vi "Open_LoopTesting_VI.vi"() -> ()   [LabVIEW 2022 SP3]
uses:
  <vilib>/DAQmx/read.llb/DAQmx Read (Analog 1D Wfm NChan NSamp).vi
  <vilib>/Analysis/baseanly.llb/Mean (DBL).vi
  STOP_GLOBAL.vi
  <vilib>/DAQmx/configure/timing.llb/DAQmx Timing (Sample Clock).vi
  <vilib>/DAQmx/miscellaneous.llb/DAQmx Fill In Error Info.vi
  <resource>/objmgr/daqmx.rc
  <vilib>/Analysis/NI_AALBase.lvlib
panel:
  out "Angle":dbl
  in  "Voltage 2":dbl
  out "Angle Sensor":dbl[](graph)
  out "Voltage Command Output":dbl[](graph)
  out "VoltageSent":dbl
  out "Ball Valve Angle Command":dynamicdata(graph)
  in  "Ignition":bool
  out "Chamber Pressure LocalVar":dynamicdata(graph)
  out "Process Variable vs Setpoint":dynamicdata(graph)
  out "Servo/Step Voltage":dbl[](array[numeric])
  in  "SP":dbl
  out "MV":dbl(slide)=30.8641975308642 scale=0.0..5.067 scale format="%.1f"
  in  "Stop All":bool
  out "D.C. Delay":dbl
  out "AI7":dynamicdata(graph)
  out "Time":dbl
  out "Inlet Thermocouple":cluster{dbl[], dbl[]}(graph)
  out "Inlet Thermocouple":dynamicdata(graph)
  out "Flow Meter Thermocouple":dynamicdata(graph)
  out "Flow Meter Thermocouple":cluster{dbl[], dbl[]}(graph)
  out "Supply P. Thermocouple":cluster{dbl[], dbl[]}(graph)
  out "Supply P. Thermocouple":dynamicdata(graph)
  out "Thrust 3":cluster{dbl[], dbl[]}(graph)
  out "Thrust 2":cluster{dbl[], dbl[]}(graph)
  out "Rocket Thrust":cluster{dbl[], dbl[]}(graph)
  out "LC2":dynamicdata(graph)
  out "Rocket Thrust LC1":dynamicdata(graph)
  out "LC3":dynamicdata(graph)
  out "Waiting \nfor Start":bool=TRUE
  in  "Start VI":bool
  out "SampClk.Rate":dbl
  in  "Sample Number":i32=100
  in  "Channel Control":bool[](array[boolean])
  in  "Rate":dbl=1000.0 format="%0.2f"
  out "AI7":cluster{dbl[], dbl[]}(graph)
  out "Vol Flow L/min":dynamicdata(graph)
  out "Chamber Pressure and Degrees":cluster{dbl[], dbl[]}[](graph)
  in  "Filename":path=path "C:/1. Rocket Research Project/CollectedData/Plots/TestingData.lvm"
  in  "Collect?":bool=TRUE caption="Enable"
  out "Vol Flow":cluster{dbl[], dbl[]}(graph)
  out "Chamber Pressure":cluster{dbl[], dbl[]}(graph)
  out "Inlet Pressure":cluster{dbl[], dbl[]}(graph)
  out "Flow Meter Pressure":cluster{dbl[], dbl[]}(graph)
  out "Supply Pressure":cluster{dbl[], dbl[]}(graph)
  out "Supply Pressure":dynamicdata(graph)
  out "Inlet Pressure":dynamicdata(graph)
  out "Line Pressure":dynamicdata(graph)
  out "Chamber Pressure PSI":dynamicdata(graph)
  out "Output Clock Rate":dbl
  out "For loop iterations":i32
  out "error out":errorcluster
  out "Iterations":i32
  out "Angle Sensor":dynamicdata(graph)
  out "P.T. 5":dynamicdata(graph)
  # "Temperature Channels"
  # "Thrust Channels"
  # "DAQ Configuration"
  # "AI 0 - Supply Pressure"
  # "AI 1 - Flow Meter Pressure"
  # "AI 2 - Inlet Pressure"
  # "AI 3 - Chamber Pressure"
  # "AI 4 - Differential Pressure"
  # "AI 5 - Volumetric Flow"
  # "AI 6 - Angle Sensor"
  # "AI 7"
  # "Load Cell 1 Right"
  # "Load Cell 2 Left"
  # "Thrust Channel 3"
  # "TC1 - Supply P. Thermocouple"
  # "TC2 - Flow Meter Thermocouple"
  # "TC3 - Inlet Thermocouple"
  # "Pressure Channels"
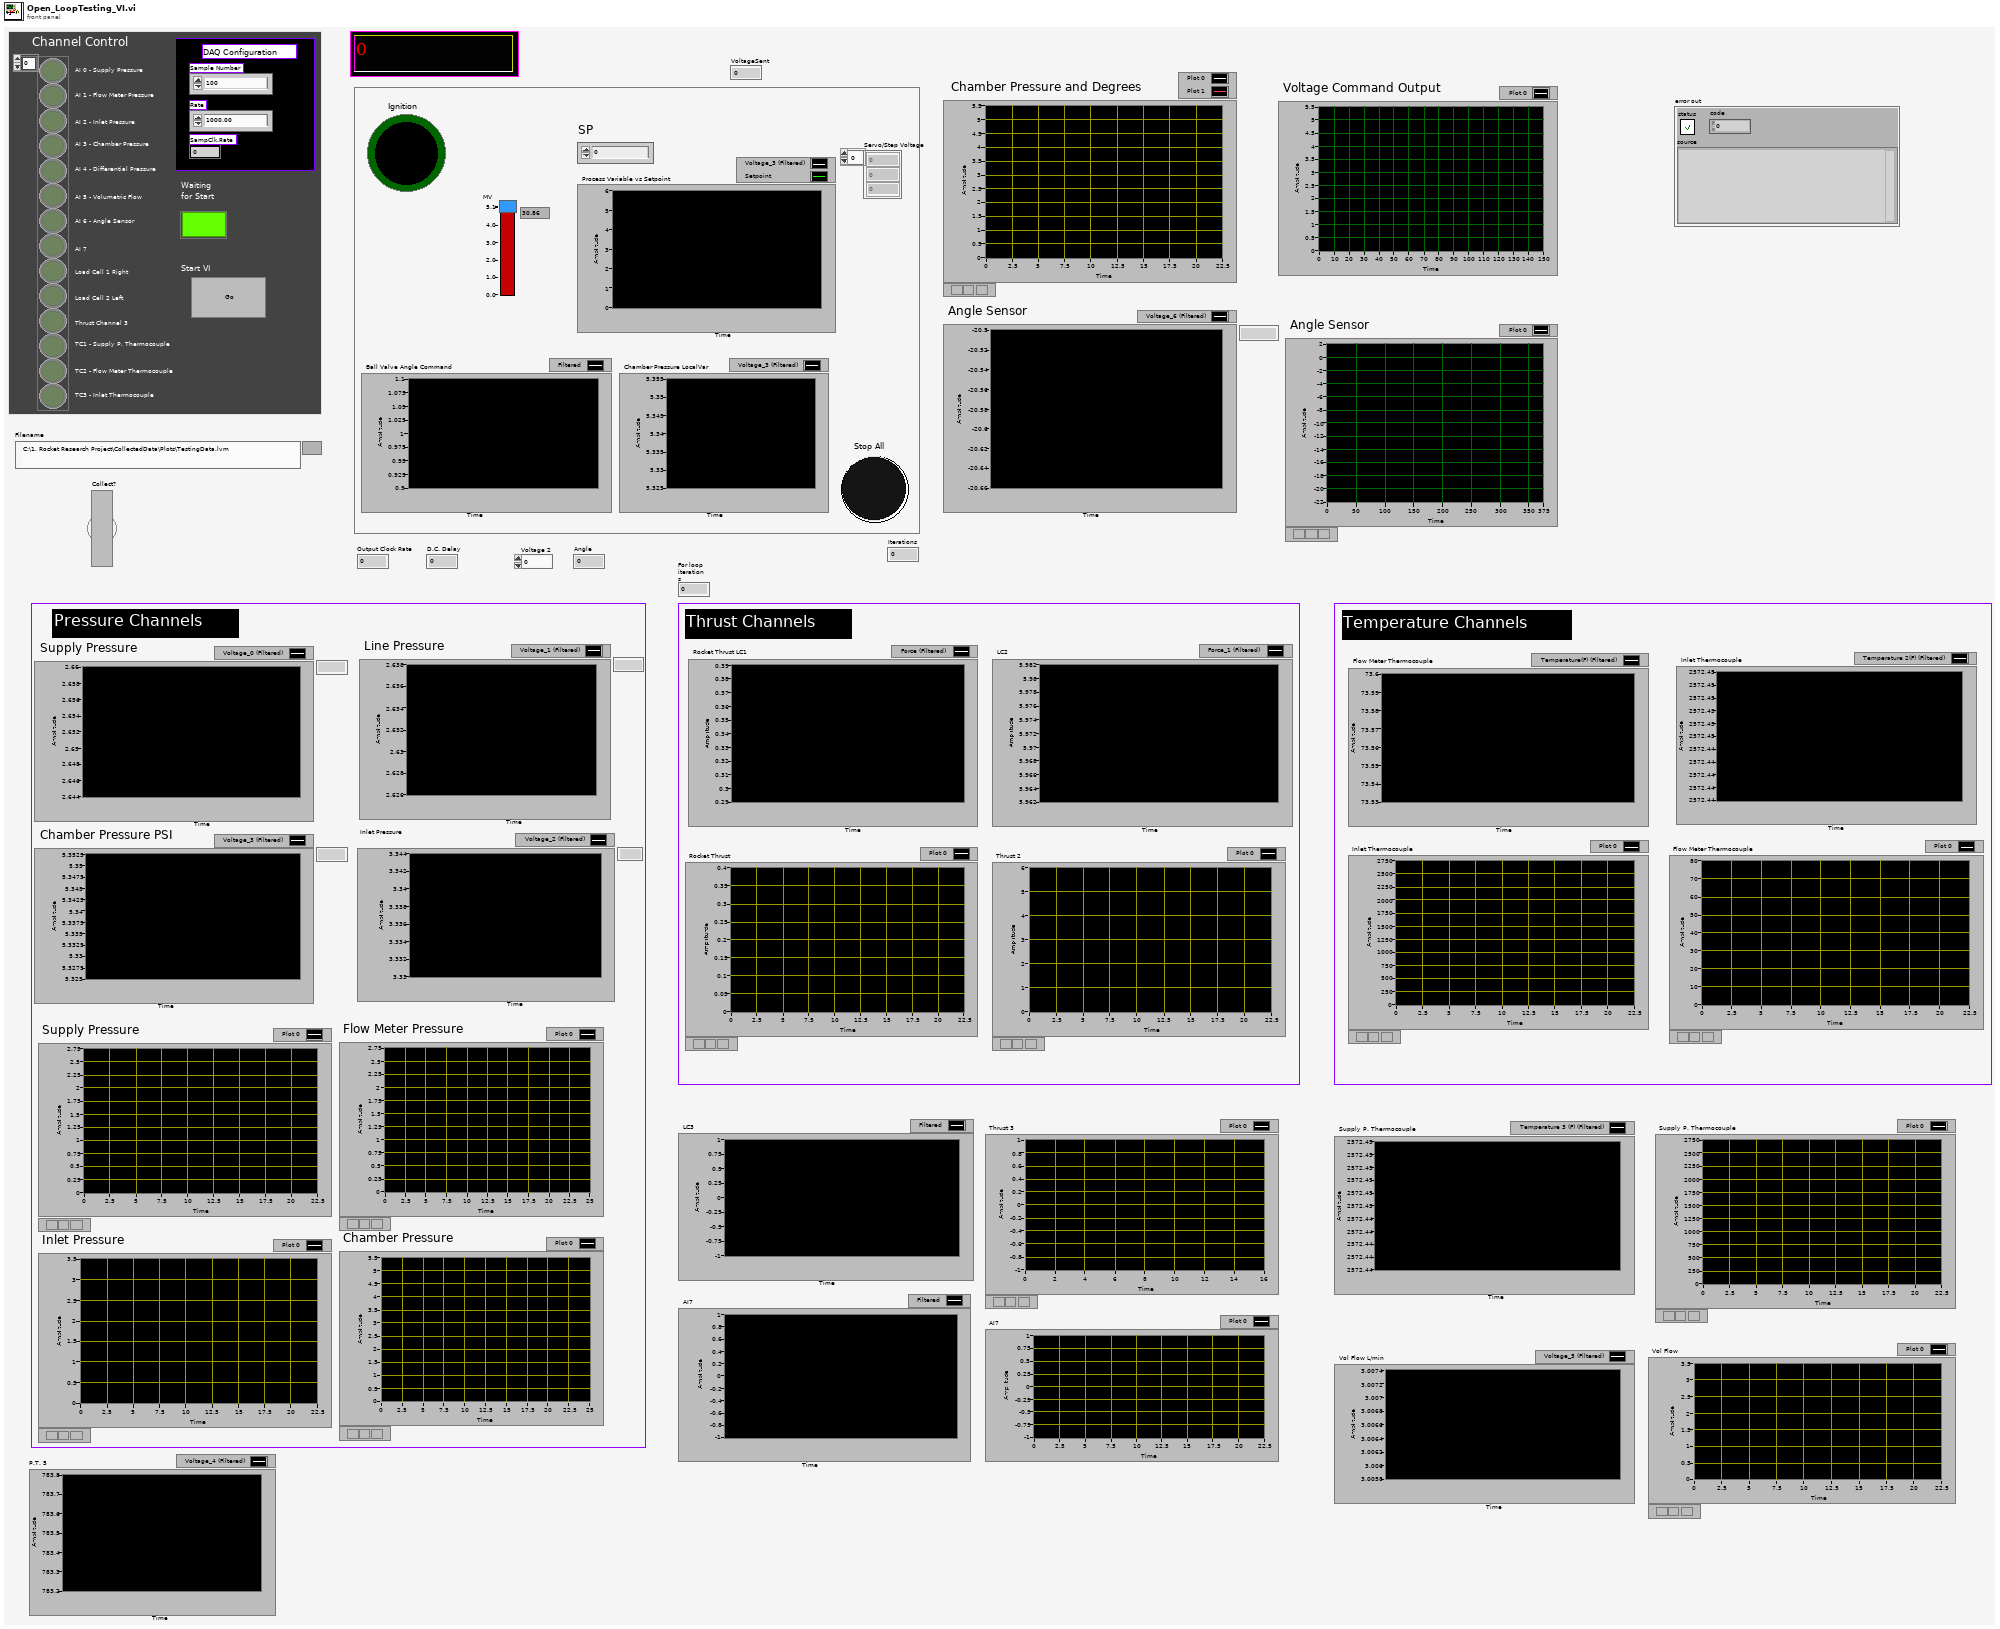
[diagram p1: front panel]
types:
  T1 = cluster{"PID gains":cluster{"Kc":dbl, "Ti":dbl, "Td":dbl}, "max value":dbl}[]
  T2 = cluster{"Modulus":dbl, "Number of\nComplete Cycles":dbl}
  T3 = cluster{"Dynamic Data":dynamicdata, "Dynamic Data":dynamicdata, "Dynamic Data":dynamicdata, "Dynamic Data":dynamicdata, "Dynamic Data":dynamicdata, "Dynamic Data":dynamicdata, "Dynamic Data":dynamicdata, "Dynamic Data":dynamicdata, "Dynamic Data":dynamicdata, "Dynamic Data":dynamicdata, "Dynamic Data":dynamicdata, "Dynamic Data":dynamicdata, "Dynamic Data":dynamicdata, "Dynamic Data":dynamicdata}
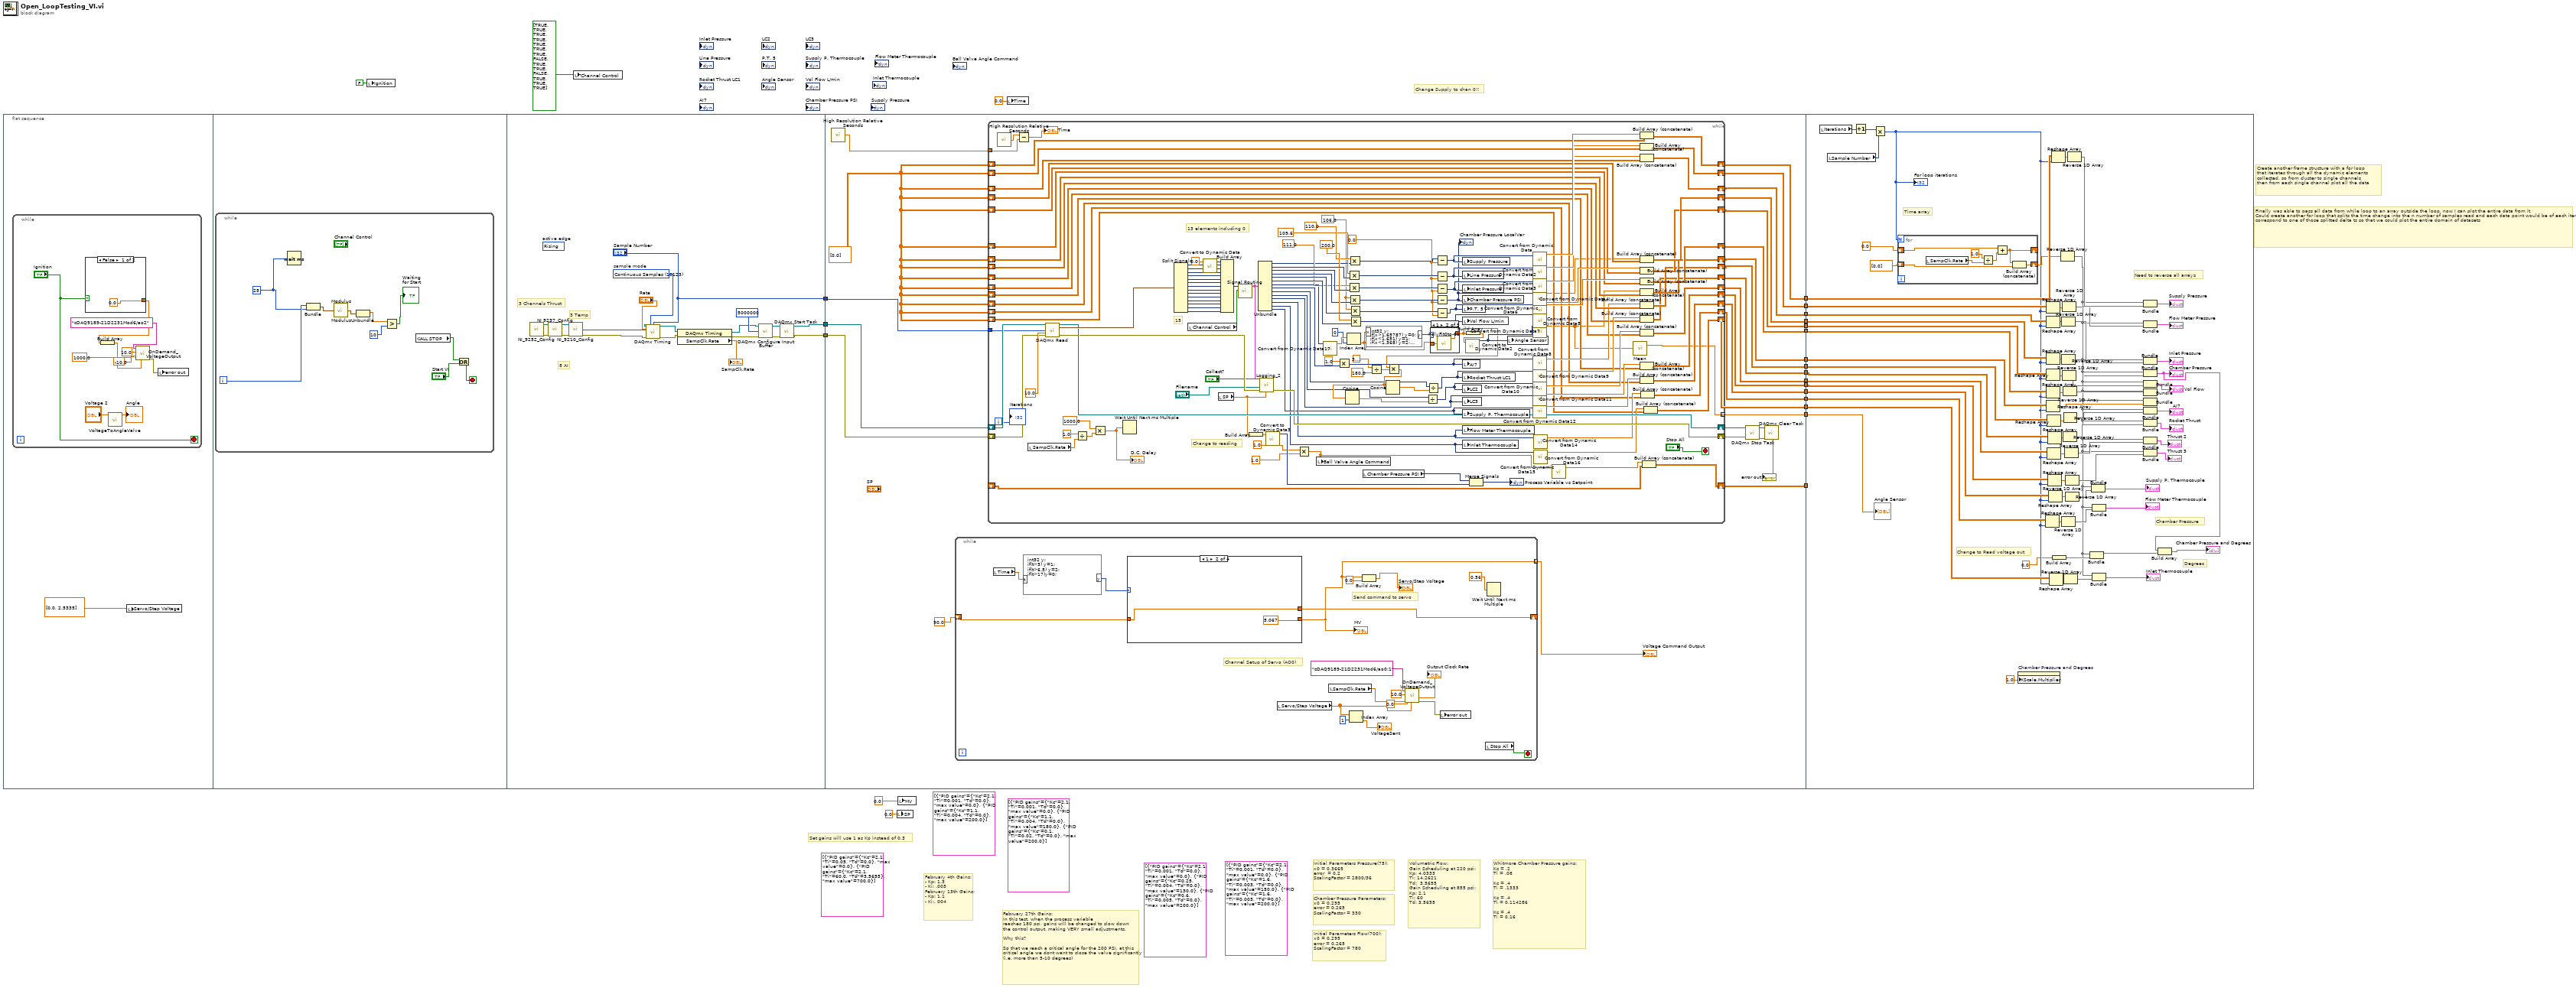
[diagram p0: block diagram]
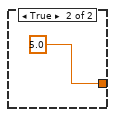
[diagram p2: hidden frame]
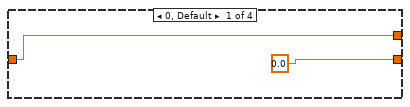
[diagram p3: hidden frame]
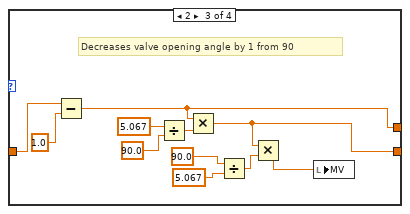
[diagram p4: hidden frame]
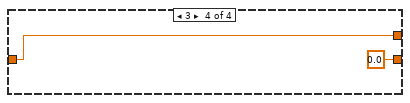
[diagram p5: hidden frame]
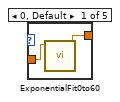
[diagram p6: hidden frame]
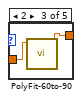
[diagram p7: hidden frame]
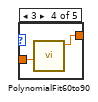
[diagram p8: hidden frame]
diagram:
  (unwired) T1 [{"PID gains"={"Kc"=2.1, "Ti"=0.001, "Td"=0.0}, "max value"=0.0}, {"PID gains"={"Kc"=1.1, "Ti"=0.004, "Td"=0.0}, "max value"=180.0}, {"PID gains"={"Kc"=0.1, "Ti"=0.02, "Td"=0.0}, "max value"=200.0}]
  (unwired) T1 [{"PID gains"={"Kc"=2.1, "Ti"=0.001, "Td"=0.0}, "max value"=0.0}, {"PID gains"={"Kc"=1.6, "Ti"=0.003, "Td"=0.0}, "max value"=150.0}, {"PID gains"={"Kc"=1.6, "Ti"=0.003, "Td"=0.0}, "max value"=200.0}]
  (unwired) T1 [{"PID gains"={"Kc"=2.1, "Ti"=0.001, "Td"=0.0}, "max value"=0.0}, {"PID gains"={"Kc"=0.25, "Ti"=0.004, "Td"=0.0}, "max value"=130.0}, {"PID gains"={"Kc"=0.6, "Ti"=0.005, "Td"=0.0}, "max value"=200.0}]
  (unwired) T1 [{"PID gains"={"Kc"=2.1, "Ti"=0.05, "Td"=0.0}, "max value"=0.0}, {"PID gains"={"Kc"=2.1, "Ti"=60.0, "Td"=3.5655}, "max value"=700.0}]
  (unwired) T1 [{"PID gains"={"Kc"=2.1, "Ti"=0.001, "Td"=0.0}, "max value"=0.0}, {"PID gains"={"Kc"=1.1, "Ti"=0.004, "Td"=0.0}, "max value"=200.0}]
  # "February 27th Gains:\nIn this test, when the process variable\nreaches 180 psi, gains will be changed to slow down\nthe control output, making VERY small adjustments.\n\nWhy this? \n\nSo that we reach a critical angle for the 200 PSI, at this\ncritical angle we dont want to close the valve significantly\n(i.e. more than 5-10 degrees)"
  # "February 4th Gains:\n- Kp: 1.3\n- Ki: .003\nFebruary 13th Gains:\n- Kp: 1.1\n- Ki:. 004"
  # "Set gains will use 1 as Kp instead of 0.3"
  # "Whitmore Chamber Pressure gains:\nKc = .2\nTi = .08\n\nKc = .4\nTi = .1333\n\nKc = .4\nTi = 0.114286\n\nKc = .4\nTi = 0.16"
  # "Chamber Pressure Parameters:\nx0 = 0.295\nerror = 0.265\nScalingFactor = 330"
  # "Volumetric Flow:\nGain Scheduling at 220 psi:\nKp: 4.0333\nTi: 14.2621\nTd:  3.5655\nGain Scheduling at 855 psi:\nKp: 2.1\nTi: 60\nTd: 3.5655"
  # "Initial Parameters Flow(700):\nx0 = 0.295\nerror = 0.265\nScalingFactor = 780"
  # "Initial Parameters Pressure(75):\nx0 = 0.3665\nerror  = 0.2\nScalingFactor = 2800/36"
  # "Change Supply to chan 0!!"
  # "Finally was able to pass all data from while loop to an array outside the loop, now I can plot the entire data from it, \nCould create another for loop that splits the time change into the n number of samples read and each data point would be of each iteration would correspond to one of those splitted delta ts so that we could plot the entire domain of datasets"
  # "Create another frame structure with a for loop\nthat iterates through all the dynamic elements\ncollected, so from cluster to single channels\nthen from each single channel plot all the data"
  n1 = flat-sequence {
    tunnel: [w59] -> w23
    tunnel: [w48] -> w22
    tunnel: ["Sample Number"] -> w4
    tunnel: w23 -> [w94]
    tunnel: w22 -> [w93]
    tunnel: [w86] -> w21
    tunnel: [w85] -> w19
    tunnel: [w84] -> w18
    tunnel: [w83] -> w17
    tunnel: [w82] -> w16
    tunnel: [w81] -> w15
    tunnel: [w80] -> w14
    tunnel: [w79] -> w13
    tunnel: [w78] -> w12
    tunnel: [w77] -> w11
    tunnel: [w76] -> w10
    tunnel: [w75] -> w9
    tunnel: [w73] -> w6
    tunnel: [w72] -> w5
    tunnel: w4 -> [w71]
    tunnel: [w70] -> w2
    tunnel: [w69] -> w1
    tunnel: w21 -> [w341]
    tunnel: w19 -> [w340]
    tunnel: w18 -> [w339]
    tunnel: w17 -> [w338]
    tunnel: w16 -> [w337]
    tunnel: w15 -> [w336]
    tunnel: w14 -> [w335]
    tunnel: w13 -> [w333]
    tunnel: w12 -> [w332]
    tunnel: w11 -> [w331]
    tunnel: w10 -> [w330]
    tunnel: w9 -> [w329]
    tunnel: w6 -> [w305]
    tunnel: w5 -> [w304]
    tunnel: w2 -> [_]
    tunnel: w1 -> [w287]
    frame #0 {
      n2 = while {
        stop <- "Ignition" stop-if-true
        n3 = case shown="False" "Ignition" {
          tunnel: [0.0 ("element") 5.0 ("element")] -> w34
          frame False {
          }
          frame True {
          }
        }
        n4 = Build Array(w34) -> (w35:dbl[])
        n5 = call "VoltageToAngleValve.vi"("Voltage"="Voltage 2") -> ("Angle"=→"Angle":dbl)  [unwired: 10 in]
        n6 = call "OnDemand_VoltageOutput.vi"("Channel Array"=w35, "SampClk.Rate 2"=1000.0, "minimum voltage"=-10.0, "maximum voltage"=10.0, "physical channels"="cDAQ9189-21D2231Mod6/ao2") -> ("error out"=w33:errorcluster)  [unwired: 4 in, 2 out]
        n7 = local write "error out"(w33) -> ()
      }
      n8 = local write "Servo/Step Voltage"(dbl[] [0.0, 2.5335] ("Servo/Step Voltage")) -> ()
    }
    frame #1 {
      n9 = while {
        i -> [w47]
        stop <- w39 stop-if-true
        w38 = u32 25 ("milliseconds to wait")
        n10 = Wait (ms)(milliseconds to wait=w38) -> ()  [unwired: 1 out]
        n11 = Bundle(w47, "milliseconds to wait"=w38) -> (w46:cluster{i32, "milliseconds to wait":u32})  [unwired: 1 in]
        n12 = call "Modulus.vi"("Input"=w46) -> ("Output"=w45:T2)
        n13 = call "Modulus.vi"() -> ()  [unwired: 1 in, 1 out]
        n14 = Unbundle(w45) -> ("Modulus"=w44:dbl)  [unwired: 1 out]
        n15 = Greater?(x=w44, y=u32 10 ("milliseconds to wait")) -> (0:→"Waiting \nfor Start":bool)
        n16 = global read "STOP_GLOBAL.vi" "ALL STOP"() -> (w41:bool)
        n17 = Or(x=w41, y="Start VI") -> (x .or. y?=w39:bool)
      }
    }
    frame #2 {
      w50 = 10123 items=["Finite Samples"=10178, "Continuous Samples"=10123, "Hardware Timed Single Point"=12522]  # sample mode
      (unwired) 10280 items=["Rising"=10280, "Falling"=10171]  # active edge
      # "3 Temp"
      # "8 AI"
      # "3 Channels Thrust"
      n18 = call "NI_9252_Config.vi"() -> ("error out"=w57:errorcluster, "task out"=w58:refnum<k21>)  [unwired: 10 in]
      n19 = call "NI 9237_Config.vi"("error in"=w57, "task in"=w58) -> ("error out"=w66:errorcluster, "task out"=w65:refnum<k21>)  [unwired: 8 in]
      n20 = call "NI_9210_Config.vi"("error in"=w66, "task in"=w65) -> ("error out"=w53:errorcluster, "task out"=w55:refnum<k21>)  [unwired: 8 in]
      n21 = call-poly <vilib>:"DAQmx Timing.vi"("task/channels in"=w55, "sample mode"=w50, "samples per channel"="Sample Number", "rate"="Rate", "error in"=w53) -> ("task out"=w51:refnum<k21>, "error out"=w52:errorcluster)  [unwired: 9 in]
      n22 = property class="DAQmx Timing"(reference=w51, error in=w52) -> (reference out=w49:refnum<k21>, error out=w62:errorcluster, "SampClk.Rate"=→"SampClk.Rate":dbl)
      n23 = call <vilib>:"DAQmx Configure Input Buffer.vi"("task/channels in"=w49, "buffer size (in samples per channel)"=u32 5000000, "error in"=w62) -> ("task out"=w64:refnum<k21>, "error out"=w63:errorcluster)  [unwired: 11 in]
      n24 = call <vilib>:"DAQmx Start Task.vi"("task/channels in"=w64, "error in"=w63) -> ("task out"=w59:refnum<k21>, "error out"=w48:errorcluster)  [unwired: 12 in]
    }
    frame #3 {
      w74 = dbl[][] [[0.0]]
      n25 = call <vilib>:"High Resolution Relative Seconds.vi"() -> ("relative seconds"=w92:dbl)
      n26 = while {
        tunnel: [w95] -> w68 mode=indexing
        shift-right: [w96] -> _
        shift-left: 90.0 -> [w97]
        stop <- w112 stop-if-true
        # "Send command to servo"
        # "Channel Setup of Servo (AO0)"
        n27 = local read "Time"() -> (w98:dbl)
        n28 = formula code="int32 y;\nif(t>3) y=1;\nif(t>6.5) y=2;\nif(t>17)y=0;"("t"=w98) -> ("y"=w100:i32)
        n29 = case shown="1" w100 {
          tunnel: [w113 w115 w119 w128] -> w96
          tunnel: w97 -> [w113 w115 w127 w128]
          tunnel: [0.0 ("MV") 5.067 ("MV") w117 0.0] -> w95
          frame 0, Default {
          }
          frame 1 {
          }
          frame 2 {
            # "Decreases valve opening angle by 1 from 90"
            n30 = Subtract(x=w127, y=1.0) -> (x-y=w119:dbl)
            n31 = Divide(x=5.067, y=90.0) -> (x/y=w125:dbl)
            n32 = Multiply(x=w119, y=w125) -> (x*y=w117:dbl)
            n33 = Divide(x=90.0 ("y"), y=5.067) -> (x/y=w121:dbl)
            n34 = Multiply(x=w117, y=w121) -> (x*y=w118:dbl)
            n35 = local write "MV"(w118) -> ()
          }
          frame 3 {
          }
        }
        "MV" <- w95
        n36 = local read "Servo/Step Voltage"() -> (w103:dbl[])
        n37 = local read "SampClk.Rate"() -> (w110:dbl)
        n38 = Index Array(array=w103, index=1) -> (element=→"VoltageSent":dbl)
        n39 = Build Array(w95, 0.0 ("element")) -> (→"Servo/Step Voltage":dbl[])
        n40 = call "OnDemand_VoltageOutput.vi"("Channel Array"=w103, "SampClk.Rate 2"=w110, "minimum voltage"=0.0, "maximum voltage"=10.0, "physical channels"="cDAQ9189-21D2231Mod6/ao0:1") -> ("error out"=w109:errorcluster, "SampClk.Rate"=→"Output Clock Rate":dbl)  [unwired: 4 in, 1 out]
        n41 = local write "error out"(w109) -> ()
        n42 = local read "Stop All"() -> (w112:bool)
        n43 = Wait Until Next ms Multiple(millisecond multiple=0.56 ("x")) -> ()  [unwired: 1 out]
      }
      "Voltage Command Output" <- w68
      n44 = while {
        shift-right: [w266] -> w88
        shift-left: w94 -> [w268]
        shift-right: [w244] -> w87
        shift-left: w93 -> [w267]
        shift-right: [w161] -> w86
        shift-left: w74 -> [w207]
        tunnel: w92 -> [w241]
        shift-right: [w236] -> w85
        shift-left: w74 -> [w133]
        shift-right: [w233] -> w84
        shift-left: w74 -> [w234]
        shift-right: [w231] -> w83
        shift-left: w74 -> [w232]
        shift-right: [w229] -> w82
        shift-left: w74 -> [w228]
        shift-right: [w226] -> w81
        shift-left: w74 -> [w224]
        shift-right: [w225] -> w80
        shift-left: w74 -> [w223]
        shift-right: [w222] -> w79
        shift-left: w74 -> [w221]
        shift-right: [w217] -> w78
        shift-left: w74 -> [w216]
        shift-right: [w215] -> w77
        shift-left: w74 -> [w214]
        shift-right: [w212] -> w76
        shift-left: w74 -> [w211]
        shift-right: [w209] -> w75
        shift-left: w74 -> [w208]
        shift-right: [w186] -> w73
        shift-left: w74 -> [w185]
        shift-right: [w182] -> w72
        shift-left: w74 -> [w183]
        tunnel: w71 -> [w179]
        shift-right: [w156] -> w70
        shift-left: _ -> [w157]
        tunnel: [w134] -> w69 mode=indexing
        i -> [w243]
        stop <- "Stop All" stop-if-true
        w155 = 106.0 ("x")
        w171 = 0.0 ("y")
        # "Change to reading"
        # "13 elements including 0"
        # "15"
        n45 = call <vilib>:"High Resolution Relative Seconds.vi"() -> ("relative seconds"=w242:dbl)
        n46 = Subtract(x=w242, y=w241) -> (x-y=→"Time":dbl)
        n47 = local read "SampClk.Rate"() -> (w204:dbl)
        n48 = call-poly <vilib>:"DAQmx Read.vi"("task/channels in"=w268, "number of samples per channel"=w179, "timeout"=10.0, "error in"=w267) -> ("task out"=w266:refnum<k21>, "data"=w269:waveform(dbl)[], "error out"=w246:errorcluster)  [unwired: 9 in]
        n49 = Divide(x=1.0, y=w204) -> (x/y=w203:dbl)
        n50 = Multiply(x=1000.0, y=w203) -> (x*y=w201:dbl)
        "D.C. Delay" <- w201
        n51 = Wait Until Next ms Multiple(millisecond multiple=w201) -> ()  [unwired: 1 out]
        n52 = Split Signals(w269) -> (w260:dynamicdata, w265:dynamicdata, w264:dynamicdata, w263:dynamicdata, w262:dynamicdata, w261:dynamicdata, w259:dynamicdata, w258:dynamicdata, w257:dynamicdata, w256:dynamicdata, w255:dynamicdata, w252:dynamicdata, w189:dynamicdata, w188:dynamicdata)  [unwired: 14 in]
        n53 = local read "Channel Control"() -> (w251:bool[])
        n54 = call "Convert to Dynamic Data"("Double"=0.0) -> ("Dynamic Data Type"=w253:dynamicdata)  [unwired: 3 in]
        n55 = local read "SP"() -> (w169:dbl)
        n56 = Build Array(w253, w260, w265, w264, w263, w262, w261, w259, w258, w257, w256, w255, w252, w189, w188) -> (w250:dynamicdata[])
        n57 = call "Signal Routing.vi"("Boolean Array"=w251, "Data In"=w250) -> ("Output"=w178:T3)  [unwired: 9 in]
        n58 = Build Array(w169) -> (w168:dbl[])
        n59 = Unbundle(w178) -> ("Dynamic Data"=w160:dynamicdata, "Dynamic Data"=w249:dynamicdata, "Dynamic Data"=w248:dynamicdata, "Dynamic Data"=w170:dynamicdata, "Dynamic Data"=w247:dynamicdata, "Dynamic Data"=w181:dynamicdata, "Dynamic Data"=w148:dynamicdata, "Dynamic Data"=w200:dynamicdata, "Dynamic Data"=w140:dynamicdata, "Dynamic Data"=w139:dynamicdata, "Dynamic Data"=w137:dynamicdata, "Dynamic Data"=w177:dynamicdata, "Dynamic Data"=w175:dynamicdata, "Dynamic Data"=w176:dynamicdata)
        n60 = call "Logging_2.vi"("Setpoint"=w169, "error in"=w246, "Filename"="Filename", "Enable"="Collect?", "output cluster"=w178) -> ("error out"=w244:errorcluster)  [unwired: 6 in]
        n61 = call "Convert to Dynamic Data3"("Array"=w168) -> ("Dynamic Data Type"=w167:dynamicdata)  [unwired: 3 in]
        n62 = Multiply(x=1.0, y=1.0) -> (x*y=w159:dbl)
        n63 = local write "Ball Valve Angle Command"(w159) -> ()
        n64 = call "Convert from Dynamic Data17"("Dynamic Data Type"=w148) -> ("Array"=w153:dbl[])  [unwired: 3 in]
        n65 = Multiply(x=1.0, y=w200) -> (x*y=w198:dynamicdata)
        n66 = Index Array(array=w153, index=0) -> (element=w136:dbl)
        n67 = Multiply(x=109.6, y=w249) -> (x*y=w196:dynamicdata)
        n68 = Multiply(x=111.0, y=w248) -> (x*y=w197:dynamicdata)
        n69 = Multiply(x=110.0, y=w160) -> (x*y=w195:dynamicdata)
        n70 = Multiply(x=w155, y=w170) -> (x*y=w191:dynamicdata)
        n71 = Multiply(x=w155, y=w247) -> (x*y=w173:dynamicdata)
        n72 = Multiply(x=200.0, y=w181) -> (x*y=w174:dynamicdata)
        n73 = local read "Chamber Pressure PSI"() -> (w165:dynamicdata)
        n74 = formula code="int32 y;\nif(x>1.65787) y=0;\nif(x<1.651) y=1;\nif(x<1.368) y=2;\nif(x>1.935) y=3;\nif(x<1.36) y=4;"("x"=w136) -> ("y"=w154:i32)
        n75 = Divide(x=3.141592653589793, y=180.0 ("x")) -> (x/y=w144:dbl)
        n76 = case shown="1" w154 {
          tunnel: w136 -> [w272 w274 w276 w278 w279]
          tunnel: [w271 w273 w275 w277 w279] -> w143
          frame 0, Default {
            n77 = call "ExponentialFit0to60.vi"("voltage"=w272) -> ("angle"=w271:dbl)  [unwired: 10 in]
          }
          frame 1 {
            n78 = call "PolyFit0to-60.vi"("input variable"=w274) -> ("output variable"=w273:dbl)  [unwired: 10 in]
          }
          frame 2 {
            n79 = call "PolyFit-60to-90.vi"("Voltage"=w276) -> ("Angle"=w275:dbl)  [unwired: 10 in]
          }
          frame 3 {
            n80 = call "PolynomialFit60to90.vi"("voltage"=w278) -> ("Angle"=w277:dbl)  [unwired: 10 in]
          }
          frame 4 {
          }
        }
        n81 = Multiply(x=w143, y=w144) -> (x*y=w142:dbl)
        n82 = Cosine(x=w142) -> (cos(x)=w149:dbl)
        n83 = Cosine(x=w142) -> (cos(x)=w150:dbl)
        n84 = Divide(x=w139, y=w149) -> (x/y=w138:dynamicdata)
        n85 = Divide(x=w140, y=w150) -> (x/y=w141:dynamicdata)
        n86 = Subtract(x=w195, y=w171) -> (x-y=w194:dynamicdata)
        n87 = Subtract(x=w196, y=w171) -> (x-y=w193:dynamicdata)
        n88 = Subtract(x=w197, y=w171) -> (x-y=w192:dynamicdata)
        n89 = Subtract(x=w191, y=w171) -> (x-y=w190:dynamicdata)
        "Chamber Pressure LocalVar" <- w190
        n90 = Subtract(x=w173, y=w171) -> (x-y=w172:dynamicdata)
        n91 = local write "Supply Pressure"(w194) -> ()
        n92 = local write "Line Pressure"(w193) -> ()
        n93 = local write "Inlet Pressure"(w192) -> ()
        n94 = local write "Chamber Pressure PSI"(w190) -> ()
        n95 = local write "P.T. 5"(w172) -> ()
        n96 = local write "Vol Flow L/min"(w174) -> ()
        n97 = local write "AI7"(w198) -> ()
        n98 = local write "Rocket Thrust LC1"(w141) -> ()
        n99 = local write "LC2"(w138) -> ()
        n100 = local write "LC3"(w137) -> ()
        n101 = local write "Supply P. Thermocouple"(w176) -> ()
        n102 = local write "Flow Meter Thermocouple"(w177) -> ()
        n103 = local write "Inlet Thermocouple"(w175) -> ()
        n104 = Build Array(w143) -> (w151:dbl[])
        n105 = call "Convert to Dynamic Data2"("Array"=w151) -> ("Dynamic Data Type"=w147:dynamicdata)  [unwired: 3 in]
        n106 = Merge Signals(w165, w167) -> (→"Process Variable vs Setpoint":dynamicdata)
        n107 = local write "Angle Sensor"(w147) -> ()
        n108 = call "Convert from Dynamic Data"("Dynamic Data Type"=w194) -> ("Array"=w240:dbl[])  [unwired: 3 in]
        n109 = call "Convert from Dynamic Data2"("Dynamic Data Type"=w193) -> ("Array"=w237:dbl[])  [unwired: 3 in]
        n110 = call "Convert from Dynamic Data3"("Dynamic Data Type"=w192) -> ("Array"=w235:dbl[])  [unwired: 3 in]
        n111 = call "Convert from Dynamic Data4"("Dynamic Data Type"=w190) -> ("Array"=w132:dbl[])  [unwired: 3 in]
        n112 = call "Convert from Dynamic Data6"("Dynamic Data Type"=w172) -> ("Array"=w227:dbl[])  [unwired: 3 in]
        n113 = call "Convert from Dynamic Data5"("Dynamic Data Type"=w174) -> ("Array"=w230:dbl[])  [unwired: 3 in]
        n114 = call "Convert from Dynamic Data7"("Dynamic Data Type"=w147) -> ("Array"=w135:dbl[])  [unwired: 3 in]
        n115 = call "Convert from Dynamic Data8"("Dynamic Data Type"=w198) -> ("Array"=w220:dbl[])  [unwired: 3 in]
        n116 = call "Convert from Dynamic Data9"("Dynamic Data Type"=w141) -> ("Array"=w219:dbl[])  [unwired: 3 in]
        n117 = call "Convert from Dynamic Data10"("Dynamic Data Type"=w138) -> ("Array"=w218:dbl[])  [unwired: 3 in]
        n118 = call "Convert from Dynamic Data11"("Dynamic Data Type"=w137) -> ("Array"=w213:dbl[])  [unwired: 3 in]
        n119 = call "Convert from Dynamic Data12"("Dynamic Data Type"=w176) -> ("Array"=w210:dbl[])  [unwired: 3 in]
        n120 = call "Convert from Dynamic Data14"("Dynamic Data Type"=w177) -> ("Array"=w187:dbl[])  [unwired: 3 in]
        n121 = call "Convert from Dynamic Data15"("Dynamic Data Type"=w175) -> ("Array"=w184:dbl[])  [unwired: 3 in]
        n122 = call "Convert from Dynamic Data16"("Dynamic Data Type"=w159) -> ("Array"=w158:dbl[])  [unwired: 3 in]
        n123 = call-poly <vilib>:"Mean.vi"("X"=w135) -> ("mean"=w134:dbl)  [unwired: 1 out]
        n124 = Build Array (concatenate)(w240, w207) -> (w161:dbl[][])
        n125 = Build Array (concatenate)(w237, w133) -> (w236:dbl[][])
        n126 = Build Array (concatenate)(w235, w234) -> (w233:dbl[][])
        n127 = Build Array (concatenate)(w132, w232) -> (w231:dbl[][])
        n128 = Build Array (concatenate)(w230, w228) -> (w229:dbl[][])
        n129 = Build Array (concatenate)(w227, w224) -> (w226:dbl[][])
        n130 = Build Array (concatenate)(w135, w223) -> (w225:dbl[][])
        n131 = Build Array (concatenate)(w220, w221) -> (w222:dbl[][])
        n132 = Build Array (concatenate)(w219, w216) -> (w217:dbl[][])
        n133 = Build Array (concatenate)(w218, w214) -> (w215:dbl[][])
        n134 = Build Array (concatenate)(w213, w211) -> (w212:dbl[][])
        n135 = Build Array (concatenate)(w210, w208) -> (w209:dbl[][])
        n136 = Build Array (concatenate)(w187, w185) -> (w186:dbl[][])
        n137 = Build Array (concatenate)(w158, w157) -> (w156:dbl[][])
        n138 = Build Array (concatenate)(w184, w183) -> (w182:dbl[][])
        "Iterations" <- w243
      }
      n139 = call <vilib>:"DAQmx Stop Task.vi"("task/channels in"=w88, "error in"=w87) -> ("task out"=w91:refnum<k21>, "error out"=w90:errorcluster)  [unwired: 12 in]
      n140 = call <vilib>:"DAQmx Clear Task.vi"("task in"=w91, "error in"=w90) -> ("error out"=→"error out":errorcluster)  [unwired: 13 in]
    }
    frame #4 {
      # "Degrees"
      # "Chamber Pressure"
      # "Change to Read voltage out"
      # "Time array"
      # "Need to reverse all arrays"
      n141 = local read "Iterations"() -> (w346:i32)
      n142 = local read "Sample Number"() -> (w289:i32)
      n143 = Increment(x=w346) -> (x+1=w345:i32)
      n144 = Multiply(x=w345, y=w289) -> (x*y=w288:i32)
      "For loop iterations" <- w288
      n145 = for {
        N: w288 -> [_]
        shift-right: [w349] -> _
        shift-left: 0.0 -> [w350]
        shift-right: [w348] -> w325
        shift-left: dbl[] [0.0] -> [w347]
        n146 = local read "SampClk.Rate"() -> (w352:dbl)
        n147 = Divide(x=1.0, y=w352) -> (x/y=w351:dbl)
        n148 = Add(x=w350, y=w351) -> (x+y=w349:dbl)
        n149 = Build Array (concatenate)(w349, w347) -> (w348:dbl[])
      }
      n150 = property on="Chamber Pressure and Degrees" class="XYGraph (strict)"("XScale.Multiplier"=1.0 ("X Scale.Offset and Multiplier:Multiplier")) -> ()  [unwired: 2 in, 2 out]
      n151 = Reshape Array(w305, w288) -> (w301:dbl[])
      n152 = Reshape Array(w340, w288) -> (w321:dbl[])
      n153 = Reshape Array(w339, w288) -> (w319:dbl[])
      n154 = Reshape Array(w338, w288) -> (w317:dbl[])
      n155 = Reshape Array(w337, w288) -> (w316:dbl[])
      n156 = Reshape Array(w336, w288) -> (w314:dbl[])
      n157 = Reshape Array(w335, w288) -> (w334:dbl[])
      n158 = Reshape Array(w333, w288) -> (w311:dbl[])
      n159 = Reshape Array(w331, w288) -> (w295:dbl[])
      n160 = Reshape Array(w332, w288) -> (w303:dbl[])
      n161 = Reshape Array(w330, w288) -> (w292:dbl[])
      n162 = Reshape Array(w329, w288) -> (w308:dbl[])
      n163 = Reshape Array(w304, w288) -> (w296:dbl[])
      n164 = Reshape Array(w341, w288) -> (w323:dbl[])
      n165 = Build Array(0.0) -> (w284:dbl[])
      n166 = Reverse 1D Array(array=w325) -> (reversed array=w282:dbl[])
      n167 = Reverse 1D Array(array=w301) -> (reversed array=w300:dbl[])
      n168 = Reverse 1D Array(array=w319) -> (reversed array=w318:dbl[])
      n169 = Reverse 1D Array(array=w317) -> (reversed array=w281:dbl[])
      n170 = Reverse 1D Array(array=w316) -> (reversed array=w315:dbl[])
      n171 = Reverse 1D Array(array=w321) -> (reversed array=w320:dbl[])
      n172 = Reverse 1D Array(array=w314) -> (reversed array=w313:dbl[])
      n173 = Reverse 1D Array(array=w303) -> (reversed array=w302:dbl[])
      n174 = Reverse 1D Array(array=w311) -> (reversed array=w310:dbl[])
      n175 = Reverse 1D Array(array=w296) -> (reversed array=w297:dbl[])
      n176 = Reverse 1D Array(array=w295) -> (reversed array=w294:dbl[])
      n177 = Reverse 1D Array(array=w292) -> (reversed array=w291:dbl[])
      n178 = Reverse 1D Array(array=w308) -> (reversed array=w307:dbl[])
      n179 = Reverse 1D Array(array=w323) -> (reversed array=w322:dbl[])
      n180 = Bundle(w282, w284) -> (w283:cluster{dbl[], dbl[]})  [unwired: 1 in]
      n181 = Bundle(w282, w307) -> (→"Supply P. Thermocouple":cluster{dbl[], dbl[]})  [unwired: 1 in]
      n182 = Bundle(w282, w300) -> (→"Flow Meter Thermocouple":cluster{dbl[], dbl[]})  [unwired: 1 in]
      n183 = Bundle(w282, w297) -> (→"Inlet Thermocouple":cluster{dbl[], dbl[]})  [unwired: 1 in]
      n184 = Bundle(w282, w322) -> (→"Supply Pressure":cluster{dbl[], dbl[]})  [unwired: 1 in]
      n185 = Bundle(w282, w320) -> (→"Flow Meter Pressure":cluster{dbl[], dbl[]})  [unwired: 1 in]
      n186 = Bundle(w282, w318) -> (→"Inlet Pressure":cluster{dbl[], dbl[]})  [unwired: 1 in]
      n187 = Bundle(w282, w281) -> (w280:cluster{dbl[], dbl[]})  [unwired: 1 in]
      "Chamber Pressure" <- w280
      n188 = Bundle(w282, w315) -> (→"Vol Flow":cluster{dbl[], dbl[]})  [unwired: 1 in]
      n189 = Bundle(w282, w313) -> ()  [unwired: 1 in, 1 out]
      n190 = Bundle(w282, w334) -> ()  [unwired: 1 in, 1 out]
      n191 = Bundle(w282, w310) -> (→"AI7":cluster{dbl[], dbl[]})  [unwired: 1 in]
      n192 = Bundle(w282, w302) -> (→"Rocket Thrust":cluster{dbl[], dbl[]})  [unwired: 1 in]
      n193 = Bundle(w282, w294) -> (→"Thrust 2":cluster{dbl[], dbl[]})  [unwired: 1 in]
      n194 = Bundle(w282, w291) -> (→"Thrust 3":cluster{dbl[], dbl[]})  [unwired: 1 in]
      n195 = Build Array(w280, w283) -> (→"Chamber Pressure and Degrees":cluster{dbl[], dbl[]}[])
      "Angle Sensor" <- w287
    }
  }
  n196 = local write "Ignition"(FALSE ("Ignition")) -> ()
  n197 = local write "Channel Control"(bool[] [TRUE, TRUE, TRUE, TRUE, TRUE, TRUE, TRUE, FALSE, TRUE, TRUE, FALSE, TRUE, TRUE, TRUE] ("Array")) -> ()
  n198 = local write "SP"(0.0 ("SP")) -> ()
  n199 = local write "MV"(0.0 ("MV")) -> ()
  n200 = local write "Time"(0.0 ("Time")) -> ()
